vi "String by Index.vi"(8 "error in (no error)":errorcluster, 10 "Index":i32, 11 "StringGroup in":refnum<class "StringGroup.lvclass">) -> (0 "error out":errorcluster, 2 "String":string, 3 "StringGroup out":refnum<class "StringGroup.lvclass">)   [LabVIEW 2020, in "Vecto.lvlib" / "StringGroup.lvclass"]
uses:
  StringGroup.lvclass
  StringGroup.lvclass/StringGroup.ctl
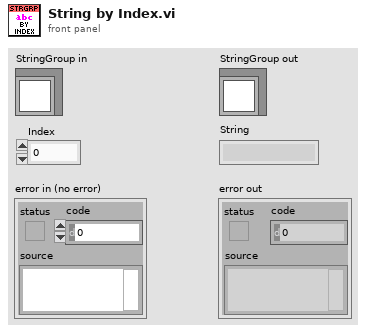
[diagram p1: front panel]
types:
  T1 = typedef "Vecto.lvlib/StringGroup.lvclass/Ref.ctl" = cluster{"Strings":string[], "Timestamp":dbl[]}
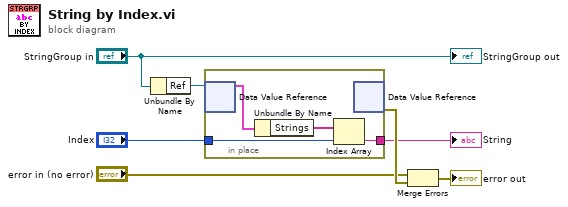
[diagram p0: block diagram]
diagram:
  n1 = Unbundle By Name("StringGroup in") -> ("Ref"=w5:refnum<data-value>)
  n2 = in-place {
    in-place-border: [w9] -> w3
    in-place-border: "Index" -> [w8]
    n3 = in-place-dvr #1(w5) -> (w11:T1)  [unwired: 1 out]
    n4 = Unbundle By Name(w11) -> ("Strings"=w10:string[])
    n5 = Index Array(array=w10, index=w8) -> (element=w9:string)
    n6 = in-place-dvr #1() -> (w7:errorcluster)  [unwired: 1 in, 1 out]
  }
  "String" <- w3
  n7 = Merge Errors("error in (no error)", w7) -> (→"error out":errorcluster)
  "StringGroup out" <- "StringGroup in"
